vi "DAQ_subvi1.vi"() -> ()   [LabVIEW 2021]
uses:
  <vilib>/DAQmx/write.llb/DAQmx Write (Digital Bool 1Line 1Point).vi
  <vilib>/DAQmx/create/channels.llb/DAQmx Create Channel (DO-Digital Output).vi
  <vilib>/DAQmx/miscellaneous.llb/DAQmx Fill In Error Info.vi
panel:
  out "error out":errorcluster
  in  "error in":errorcluster
  in  "Channel":i32
  in  "auto start 2":bool=TRUE
  in  "ON/OFF":bool=TRUE
  out "task out 2":refnum<k21>
  in  "All OFF":bool
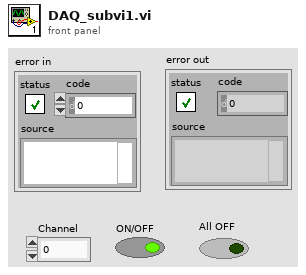
[diagram p1: front panel]
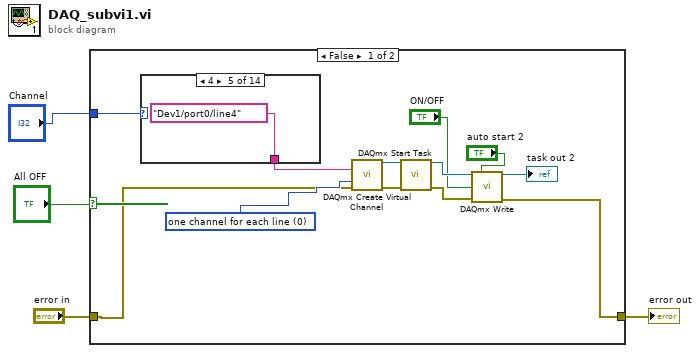
[diagram p0: block diagram]
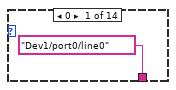
[diagram p2: hidden frame]
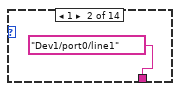
[diagram p3: hidden frame]
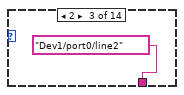
[diagram p4: hidden frame]
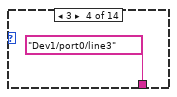
[diagram p5: hidden frame]
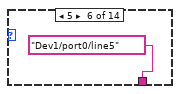
[diagram p6: hidden frame]
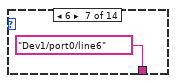
[diagram p7: hidden frame]
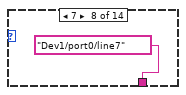
[diagram p8: hidden frame]
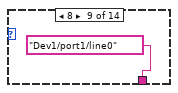
[diagram p9: hidden frame]
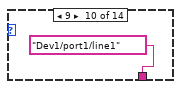
[diagram p10: hidden frame]
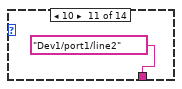
[diagram p11: hidden frame]
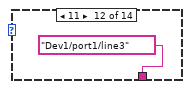
[diagram p12: hidden frame]
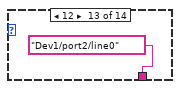
[diagram p13: hidden frame]
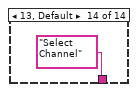
[diagram p14: hidden frame]
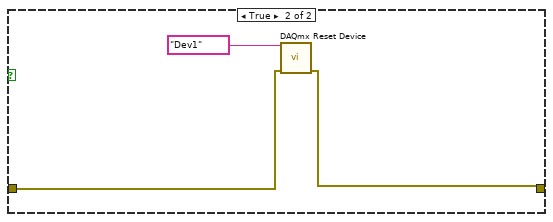
[diagram p15: hidden frame]
diagram:
  n1 = case shown="False" "All OFF" {
    tunnel: "Channel" -> [w9 _]
    tunnel: "error in" -> [w8 w32]
    tunnel: [w5 w31] -> w1
    frame False {
      w13 = 0 items=["one channel for each line", "one channel for all lines"] ("line grouping")
      n2 = case shown="4" w9 {
        tunnel: [tag "Dev1/port0/line0" ("lines") tag "Dev1/port0/line1" ("lines 2") tag "Dev1/port0/line2" ("lines 2") tag "Dev1/port0/line3" ("lines 2") tag "Dev1/port0/line4" ("lines 2") tag "Dev1/port0/line5" ("lines 2") tag "Dev1/port0/line6" ("lines 2") tag "Dev1/port0/line7" ("lines 2") tag "Dev1/port1/line0" ("lines 2") tag "Dev1/port1/line1" ("lines 2") tag "Dev1/port1/line2" ("lines 2") tag "Dev1/port1/line3" ("lines 2") tag "Dev1/port2/line0" ("lines 2") "Select Channel"] -> w10
        frame 0 {
        }
        frame 1 {
        }
        frame 2 {
        }
        frame 3 {
        }
        frame 4 {
        }
        frame 5 {
        }
        frame 6 {
        }
        frame 7 {
        }
        frame 8 {
        }
        frame 9 {
        }
        frame 10 {
        }
        frame 11 {
        }
        frame 12 {
        }
        frame 13, Default {
        }
      }
      n3 = call-poly <vilib>:"DAQmx Create Virtual Channel.vi"("lines"=w10, "line grouping"=w13, "error in"=w8) -> ("task out"=w12:refnum<k21>, "error out"=w7:errorcluster)  [unwired: 11 in]
      n4 = call <vilib>:"DAQmx Start Task.vi"("task/channels in"=w12, "error in"=w7) -> ("task out"=w15:refnum<k21>, "error out"=w6:errorcluster)  [unwired: 12 in]
      n5 = call-poly <vilib>:"DAQmx Write.vi"("task/channels in"=w15, "auto start"="auto start 2", "data"="ON/OFF", "error in"=w6) -> ("task out"=→"task out 2":refnum<k21>, "error out"=w5:errorcluster)  [unwired: 9 in, 1 out]
    }
    frame True {
      n6 = call <vilib>:"DAQmx Reset Device.vi"("device in"=tag "Dev1", "error in"=w32) -> ("error out"=w31:errorcluster)  [unwired: 13 in]
    }
  }
  "error out" <- w1
